vi "Configure Arbitrary Waveform.vi"(4 "Frequency (1000 Hz)":dbl=1000.0, 6 "Offset (0.00 V)":dbl, 8 "error in (no error)":errorcluster, 9 "Gain (1.0)":dbl=1.0, 10 "Arbitrary Waveform Name (\"ARB1\")":string="ARB1", 11 "VISA resource name":refnum<visa-resource-name>) -> (0 "error out":errorcluster, 3 "VISA resource name out":refnum<visa-resource-name>)   [LabVIEW 2020, in "Agilent 33XXX Series.lvlib"]
doc: "This VI will set the waveform parameters for an arbitrary waveform and make it the active waveform function. It should be called after Create Arbitrary Waveform."
uses:
  Agilent 33XXX Series.lvlib
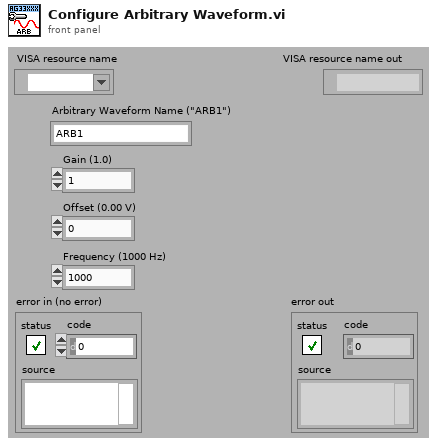
[diagram p1: front panel]
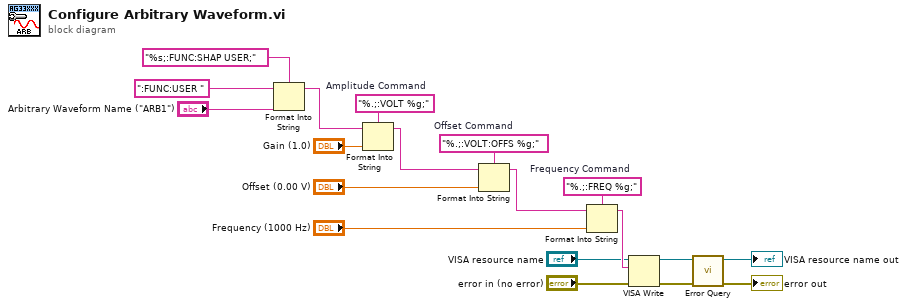
[diagram p0: block diagram]
diagram:
  w17 = "%.;:VOLT:OFFS %g;"  # Offset Command
  w18 = "%.;:VOLT %g;"  # Amplitude Command
  w19 = "%.;:FREQ %g;"  # Frequency Command
  n1 = Format Into String(format string="%s;:FUNC:SHAP USER;", initial string=":FUNC:USER ", "Arbitrary Waveform Name (\"ARB1\")") -> (resulting string=w5:string)  [unwired: 1 in, 1 out]
  n2 = Format Into String(format string=w18, initial string=w5, "Gain (1.0)") -> (resulting string=w13:string)  [unwired: 1 in, 1 out]
  n3 = Format Into String(format string=w17, initial string=w13, "Offset (0.00 V)") -> (resulting string=w12:string)  [unwired: 1 in, 1 out]
  n4 = Format Into String(format string=w19, initial string=w12, "Frequency (1000 Hz)") -> (resulting string=w11:string)  [unwired: 1 in, 1 out]
  n5 = VISA Write(VISA resource name="VISA resource name", write buffer=w11, error in (no error)="error in (no error)") -> (VISA resource name out=w10:refnum<visa-resource-name>, error out=w9:errorcluster)  [unwired: 1 out]
  n6 = call "Error Query.vi"("error in (no error)"=w9, "VISA resource name"=w10) -> ("error out"=→"error out":errorcluster, "VISA resource name out"=→"VISA resource name out":refnum<visa-resource-name>)  [unwired: 6 in, 2 out]
